vi "Read A.vi"(8 "error in (no error)":errorcluster, 11 "StateFunction in":refnum<class "StateFunction.lvclass">) -> (0 "error out":errorcluster, 2 "A":dbl[][][](array[numeric]), 3 "StateFunction out":refnum<class "StateFunction.lvclass">)   [LabVIEW 2014, in "StateFunction.lvclass"]
uses:
  StateFunction.lvclass
  StateFunction.lvclass/StateFunction.ctl
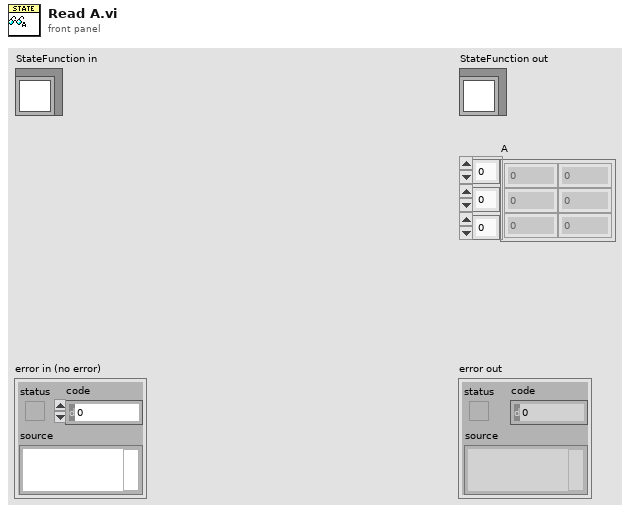
[diagram p1: front panel]
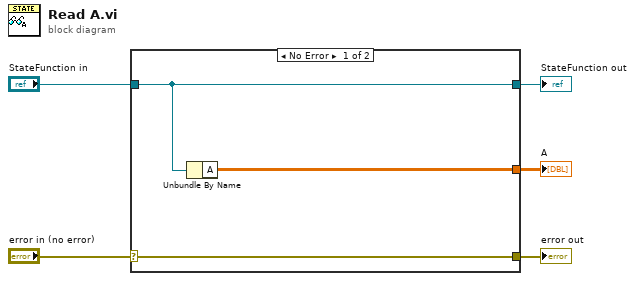
[diagram p0: block diagram]
diagram:
  n1 = case shown="No Error" "error in (no error)" {
    selector: "error in (no error)" -> [w8 w9]
    tunnel: [w8 w9] -> w4
    tunnel: [w7 w10] -> w2
    tunnel: "StateFunction in" -> [w7 w10]
    tunnel: [w6 _] -> w1
    frame No Error {
      n2 = Unbundle By Name(w7) -> ("A"=w6:dbl[][][])
    }
    frame Error {
    }
  }
  "error out" <- w4
  "StateFunction out" <- w2
  "A" <- w1
